vi "Edit-settings.vi"(8 "error in (no error)":errorcluster, 11 "Reference in":T3) -> (0 "error out":errorcluster, 3 "Reference out":T3)   [LabVIEW 2013, in "MaterialCharacterization.lvlib" / "MC-ScanParser.lvclass"]
uses:
  MC-ScanParser.lvclass
  Object-reference.ctl
  Field-properties.ctl
  Laser-properties.ctl
  MC-ScanParser.lvclass/MC-ScanParser.ctl
panel:
  in  "Cancel":bool
  in  "Ok":bool
  in  "Laser properties":T1={"MaximumLaserPower"=500.0, "Power curve"={"Watt"=[0.0, 500.0], "Bits"=[0, 255]}, "Rise time"=10, "Fall time"=10}
  in  "Field properties":T2={"Layer height"=0.05000000074505806, "MaximumFieldWidth"=0.0, "MaximumFieldHeight"=0.0, "MaximumFieldRadius"=40.0, "MaxAcceleration"=10000000.0, "MaxMarkSpeed"=10000.0, "MaxJumpSpeed"=10000.0}
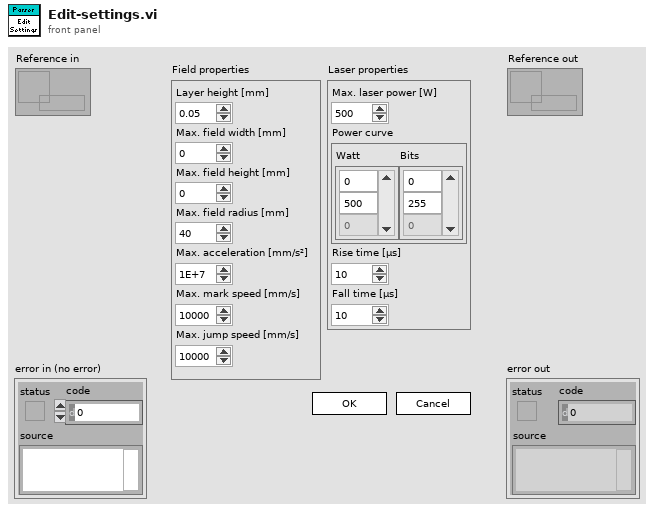
[diagram p1: front panel]
types:
  T1 = typedef "MaterialCharacterization.lvlib/MC-ScanParser.lvclass/Laser-properties.ctl" = cluster{"MaximumLaserPower":dbl, "Power curve":cluster{"Watt":dbl[], "Bits":u8[]}, "Rise time":i64, "Fall time":i64}
  T2 = typedef "MaterialCharacterization.lvlib/MC-ScanParser.lvclass/Field-properties.ctl" = cluster{"Layer height":dbl, "MaximumFieldWidth":dbl, "MaximumFieldHeight":dbl, "MaximumFieldRadius":dbl, "MaxAcceleration":dbl, "MaxMarkSpeed":dbl, "MaxJumpSpeed":dbl}
  T3 = typedef "MaterialCharacterization.lvlib/MC-ScanParser.lvclass/Object-reference.ctl" = refnum<data-value>
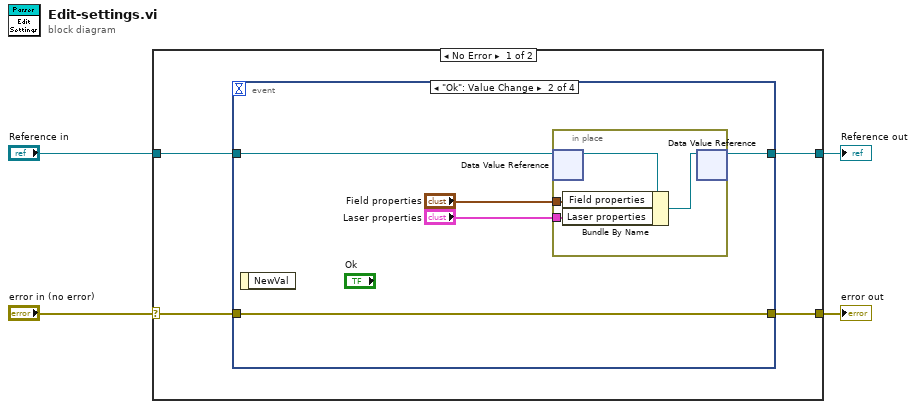
[diagram p0: block diagram]
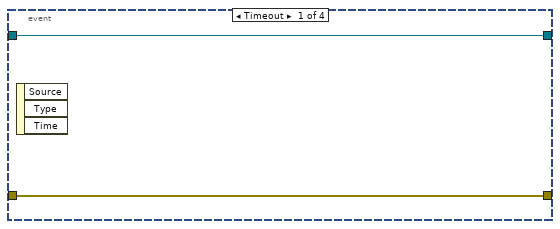
[diagram p2: hidden frame]
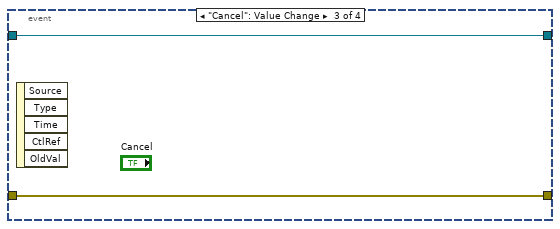
[diagram p3: hidden frame]
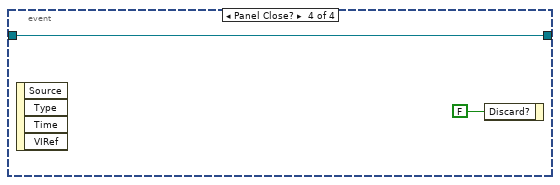
[diagram p4: hidden frame]
diagram:
  n1 = case shown="No Error" "error in (no error)" {
    selector: "error in (no error)" -> [w8 w24]
    tunnel: [w5 w24] -> w3
    tunnel: [w6 w25] -> w1
    tunnel: "Reference in" -> [w7 w25]
    frame No Error {
      n2 = event shown="[1] \"Ok\": Value Change" {
        selector: _ -> [_ _ _ _]
        dyn-events: _ -> [_ _ _ _]
        timeout: _ -> [_ _ _ _]
        tunnel: w8 -> [w10 w11 w21 _]
        tunnel: w7 -> [w9 w15 w20 w22]
        tunnel: [w9 w14 w20 w22] -> w6
        tunnel: [w10 w11 w21 _] -> w5
        event Timeout {
          n3 = event-data() -> ()  [unwired: 1 in, 3 out]
        }
        event "Ok": Value Change {
          n4 = event-data() -> ()  [unwired: 1 in, 1 out]
          n5 = in-place {
            in-place-border: "Field properties" -> [w17]
            in-place-border: "Laser properties" -> [w16]
            n6 = in-place-dvr #1(w15) -> (w19:refnum<class "MC-ScanParser.lvclass">)  [unwired: 1 out]
            n7 = Bundle By Name(cluster=w19, "Field properties"=w17, "Laser properties"=w16) -> (w18:refnum<class "MC-ScanParser.lvclass">)
            n8 = in-place-dvr #1(w18) -> (w14:T3)  [unwired: 1 out]
          }
        }
        event "Cancel": Value Change {
          n9 = event-data() -> ()  [unwired: 1 in, 5 out]
        }
        event Panel Close? {
          n10 = event-data() -> ()  [unwired: 1 in, 4 out]
          n11 = event-data("Discard?"=FALSE) -> ()  [unwired: 1 in, 1 out]
        }
      }
    }
    frame Error {
    }
  }
  "error out" <- w3
  "Reference out" <- w1
